vi "CreateManyFolders.vi"(4 "error in":errorcluster, 6 "NumFiles":i32=100, 7 "Folder name":string) -> (0 "error out":errorcluster, 2 "Elapsed Time (ms)":u32, 3 "created path":path)   [LabVIEW 2017]
panel:
  # "Creates subdirectory of home"
  # "Creates this many empty subfolders in that directory"
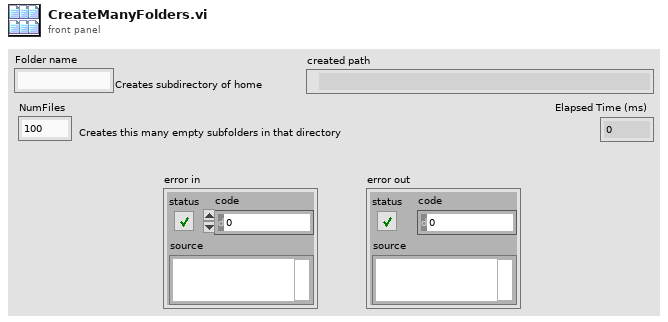
[diagram p1: front panel]
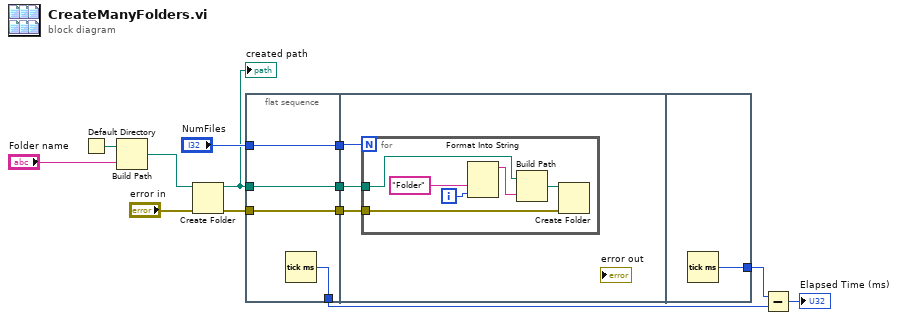
[diagram p0: block diagram]
diagram:
  n1 = Default Directory() -> (w13:path)
  n2 = Build Path(base path=w13, name or relative path="Folder name") -> (appended path=w9:path)
  n3 = Create Folder(path (use dialog)=w9, error in="error in") -> (created path=w10:path, error out=w7:errorcluster)  [unwired: 1 in, 1 out]
  "created path" <- w10
  n4 = flat-sequence {
    tunnel: w7 -> [w15]
    tunnel: w10 -> [w16]
    tunnel: "NumFiles" -> [w17]
    tunnel: [w17] -> w6
    tunnel: [w16] -> w5
    tunnel: [w15] -> w4
    tunnel: [w14] -> w1
    tunnel: w6 -> [w20]
    tunnel: w5 -> [w19]
    tunnel: w4 -> [w18]
    tunnel: [w27] -> w2
    frame #0 {
      n5 = Tick Count (ms)() -> (millisecond timer value=w14:u32)
    }
    frame #1 {
      n6 = for {
        N: w20 -> [_]
        tunnel: w19 -> [w26]
        tunnel: w18 -> [w24]
        i -> [w22]
        n7 = Format Into String("Folder", w22) -> (resulting string=w23:string)  [unwired: 3 in, 1 out]
        n8 = Build Path(base path=w26, name or relative path=w23) -> (appended path=w25:path)
        n9 = Create Folder(path (use dialog)=w25, error in=w24) -> ()  [unwired: 1 in, 3 out]
      }
    }
    frame #2 {
      n10 = Tick Count (ms)() -> (millisecond timer value=w27:u32)
    }
  }
  n11 = Subtract(x=w2, y=w1) -> (x-y=→"Elapsed Time (ms)":u32)
